vi "sqrx.vi"() -> ()   [LabVIEW 2022 SP3]
uses:
  <instrlib>/niUSRP/niUSRP Fetch Rx Data (CDB WDT).vi
panel:
  out "Waveform Graph":dynamicdata(graph)
  in  "device names":refnum<k15>
  out "error out":errorcluster
  in  "active antenna":string
  in  "gain":dbl format="%#_6f"
  in  "carrier frequency":dbl=100000.0 format="%#_6p"
  in  "IQ rate":dbl=100000.0 format="%#_6p"
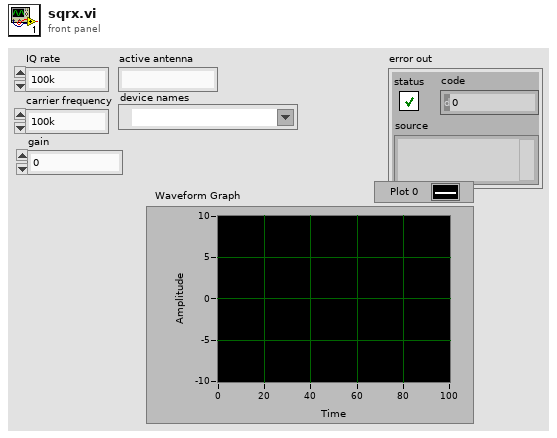
[diagram p1: front panel]
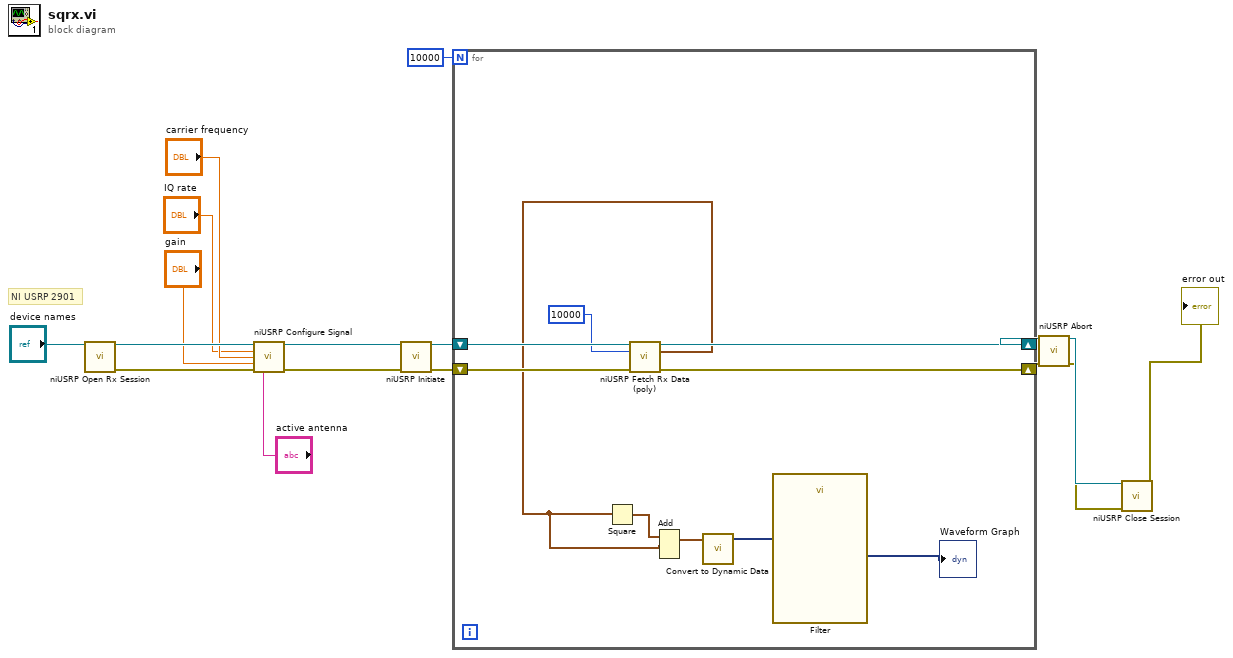
[diagram p0: block diagram]
diagram:
  # "NI USRP 2901"
  n1 = call <instrlib>:"niUSRP Open Rx Session.vi"("device names"="device names") -> ("session handle out"=w14:refnum<k15>, "error out"=w13:errorcluster)  [unwired: 13 in]
  n2 = call <instrlib>:"niUSRP Configure Signal.vi"("session handle"=w14, "IQ rate"="IQ rate", "carrier frequency"="carrier frequency", "gain"="gain", "error in (no error)"=w13, "active antenna"="active antenna") -> ("session handle out"=w12:refnum<k15>, "error out"=w15:errorcluster)  [unwired: 5 in, 3 out]
  n3 = call <instrlib>:"niUSRP Initiate.vi"("session handle"=w12, "error in (no error)"=w15) -> ("session handle out"=w5:refnum<k15>, "error out"=w4:errorcluster)  [unwired: 12 in]
  n4 = for {
    N: 10000 -> [_]
    shift-right: [w25] -> w3
    shift-left: w5 -> [w27]
    shift-right: [w24] -> w2
    shift-left: w4 -> [w26]
    n5 = call-poly <instrlib>:"niUSRP Fetch Rx Data (poly).vi"("session handle"=w27, "number of samples"=10000, "error in (no error)"=w26) -> ("session handle out"=w25:refnum<k15>, "data"=w19:waveform(cdb), "error out"=w24:errorcluster)  [unwired: 9 in, 1 out]
    n6 = Square(x=w19) -> (x^2=w23:waveform(cdb))
    n7 = Add(1:w19, 2:w23) -> (0:w22:waveform(cdb))  [unwired: 1 in, 1 out]
    n8 = call "Convert to Dynamic Data"("Waveform"=w22) -> ("Dynamic Data Type"=w21:dynamicdata)  [unwired: 3 in]
    n9 = call "Filter"("Signal"=w21) -> ("Filtered Signal"=→"Waveform Graph":dynamicdata)  [unwired: 9 in, 1 out]
  }
  n10 = call <instrlib>:"niUSRP Abort.vi"("session handle"=w3, "error in (no error)"=w2) -> ("session handle out"=w17:refnum<k15>, "error out"=w16:errorcluster)  [unwired: 12 in]
  n11 = call <instrlib>:"niUSRP Close Session.vi"("session handle"=w17, "error in (no error)"=w16) -> ("error out"=→"error out":errorcluster)  [unwired: 13 in]
